vi "DllTest.vi"() -> ()   [LabVIEW 2023]
uses:
  D:/Projects/S7View/S7Lib/bin/Debug/S7Lib.dll
  S7Lib/bin/Debug/S7Lib.dll
panel:
  in  "bit 2":u8
  in  "start 6":u16
  out "IsRunning":bool
  in  "trim":bool
  out "字符串 3":string="|"
  in  "size 3":u16=20
  in  "start 5":u16=42
  out "R_DB_Bits 2":bool[](array[boolean])
  in  "start 4":u16
  in  "count 2":u16
  out "R_DB_Bits":bool[](array[boolean])
  in  "bit":u8
  in  "count":u16
  out "字符串 2":string="|"
  in  "size 2":u16=20
  in  "start 3":u16=40
  in  "start 2":u16=62
  in  "size":u16=20
  out "字符串":string="|"
  out "R_DB_Floats":sgl[](array[numeric])
  in  "start":u16
  in  "db":u16=6000
  out "错误输出":errorcluster
  in  "布尔":bool
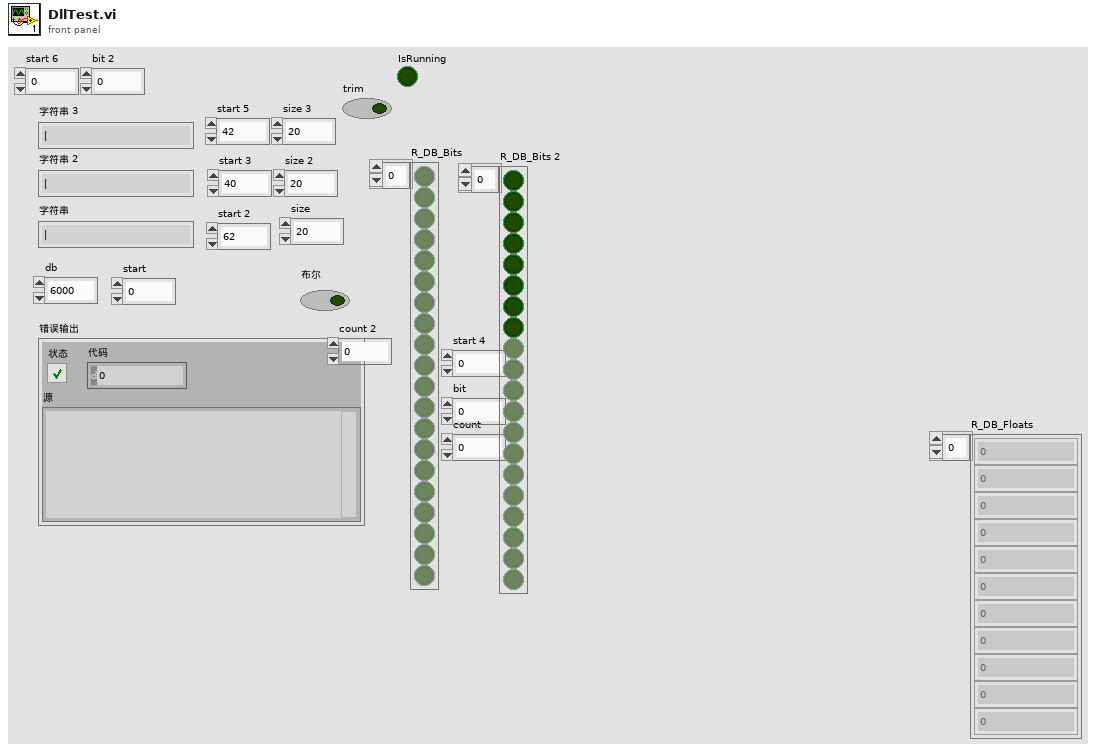
[diagram p1: front panel]
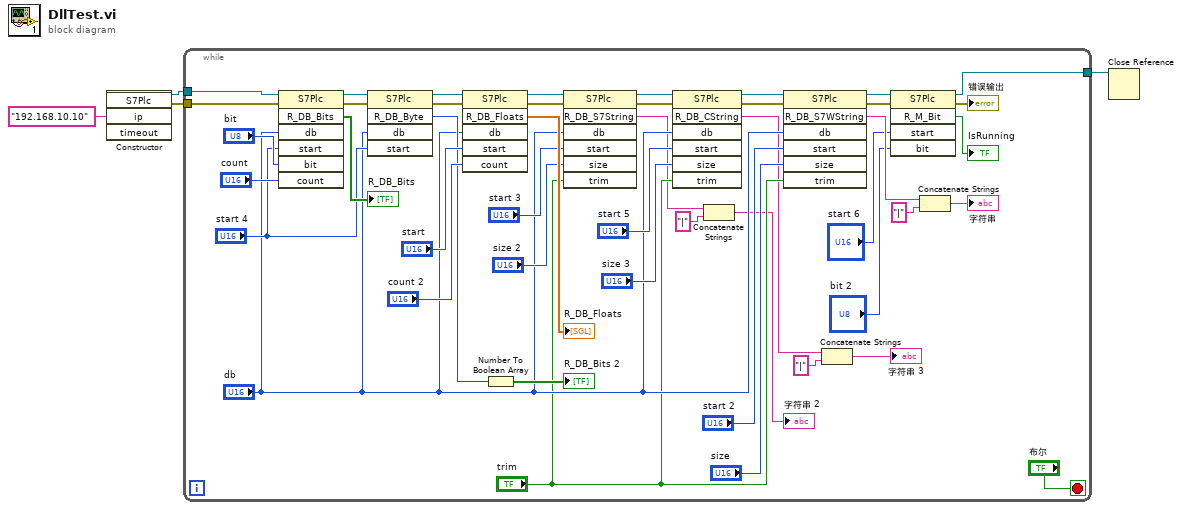
[diagram p0: block diagram]
diagram:
  n1 = constructor class="S7Plc"("ip"="192.168.10.10") -> (reference out=w4:refnum<k24>, error out=w3:errorcluster)  [unwired: 4 in, 3 out]
  n2 = while {
    tunnel: w4 -> [w12]
    tunnel: w3 -> [w50]
    tunnel: [w7] -> w1
    stop <- "布尔" stop-if-true
    n3 = invoke on="调用节点" class="S7Plc" method="R_DB_Bits"(reference=w12, error in=w50, "db"="db", "start"="start 4", "bit"="bit", "count"="count") -> (reference out=w31:refnum<k24>, error out=w33:errorcluster, "R_DB_Bits"=→"R_DB_Bits":bool[])  [unwired: 1 in, 4 out]
    n4 = invoke on="调用节点" class="S7Plc" method="R_DB_Byte"(reference=w31, error in=w33, "db"="db", "start"="start 4") -> (reference out=w30:refnum<k24>, error out=w32:errorcluster, "R_DB_Byte"=w36:u8)  [unwired: 1 in, 2 out]
    n5 = invoke on="调用节点" class="S7Plc" method="R_DB_Floats"(reference=w30, error in=w32, "db"="db", "start"="start", "count"="count 2") -> (reference out=w44:refnum<k24>, error out=w43:errorcluster, "R_DB_Floats"=→"R_DB_Floats":sgl[])  [unwired: 1 in, 3 out]
    n6 = Number To Boolean Array(number=w36) -> (Boolean array=→"R_DB_Bits 2":bool[])
    n7 = invoke on="调用节点" class="S7Plc" method="R_DB_S7String"(reference=w44, error in=w43, "db"="db", "start"="start 3", "size"="size 2", "trim"="trim") -> (reference out=w25:refnum<k24>, error out=w27:errorcluster, "R_DB_S7String"=w14:string)  [unwired: 1 in, 4 out]
    n8 = invoke on="调用节点" class="S7Plc" method="R_DB_CString"(reference=w25, error in=w27, "db"="db", "start"="start 5", "size"="size 3", "trim"="trim") -> (reference out=w24:refnum<k24>, error out=w26:errorcluster, "R_DB_CString"=w17:string)  [unwired: 1 in, 4 out]
    n9 = Concatenate Strings(w14, "|" ("字符串")) -> (→"字符串 2":string)
    n10 = invoke on="调用节点" class="S7Plc" method="R_DB_S7WString"(reference=w24, error in=w26, "db"="db", "start"="start 2", "size"="size", "trim"="trim") -> (reference out=w8:refnum<k24>, error out=w5:errorcluster, "R_DB_S7WString"=w21:string)  [unwired: 1 in, 4 out]
    n11 = Concatenate Strings(w17, "|" ("字符串")) -> (→"字符串 3":string)
    n12 = invoke on="调用节点" class="S7Plc" method="R_M_Bit"(reference=w8, error in=w5, "start"="start 6", "bit"="bit 2") -> (reference out=w7:refnum<k24>, error out=→"错误输出":errorcluster, "R_M_Bit"=→"IsRunning":bool)  [unwired: 1 in, 2 out]
    n13 = Concatenate Strings(w21, "|" ("字符串")) -> (→"字符串":string)
  }
  n14 = Close Reference(reference=w1) -> ()  [unwired: 1 in, 1 out]
